vi "ClientGlobalVariables.vi"() -> ()   [LabVIEW 2025]
panel:
  out "ID":u32
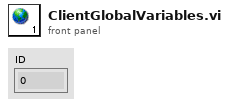
[diagram p1: front panel]
diagram:
